vi "Deserialisierer.vi"(9 "Enum":T3(ring), 11 "CAN Daten":T1[](array[typedef]) {"payload" format="%x"; "timestamp" format="%<%.7X\n%x>T"; "type" items=["CAN Data"=0, "CAN Remote"=1, "CAN Bus Error"=2, "CAN 2.0 Data"=8, "CAN FD Data"=16, "CAN FD+BRS Data"=24, "J1939 Data"=192, "Delay"=224, "Log Trigger"=225, "Start Trigger"=226]; "identifier" format="%x"}) -> (1 "Output":sgl[](array[numeric]), 3 "identifier":u32)   [LabVIEW 2020, in "CAN Interface.lvlib"]
uses:
  CAN Interface.lvlib
  <vilib>/xnet/xnet.llb/XNET Frame CAN.ctl
  <vilib>/xnet/xnet.llb/XNET Frame Type CAN.ctl
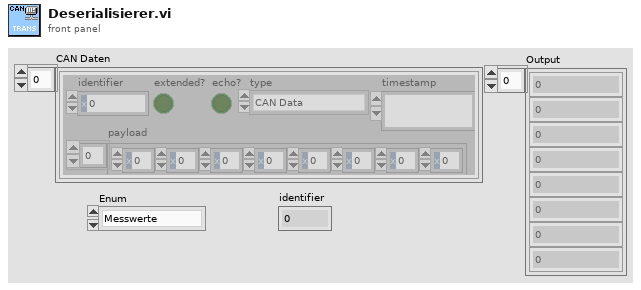
[diagram p1: front panel]
types:
  T1 = typedef "XNET Frame CAN.ctl" = cluster{"timestamp":timestamp, "payload":u8[], "identifier":u32, "type":T2, "extended?":bool, "echo?":bool}
  T2 = typedef "XNET Frame Type CAN.ctl" = u8
  T3 = enum16{"Messwerte", "Fluss, Druck", "Temperaturen 1", "Temperaturen 2", "Fehler", "Zustand, spülen?"}
  T4 = enum16{"big-endian, network order", "native, host order", "little-endian"}
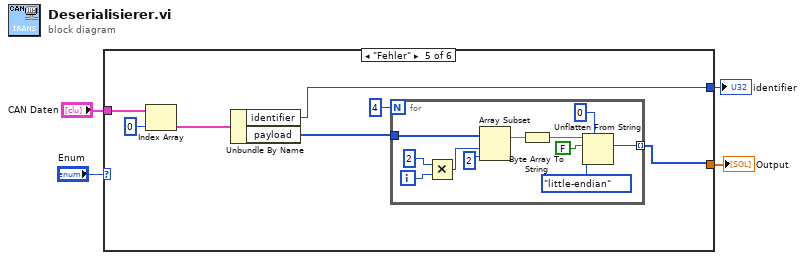
[diagram p0: block diagram]
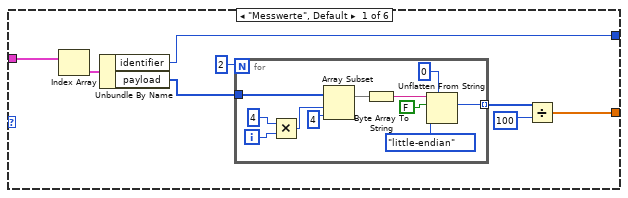
[diagram p2: hidden frame]
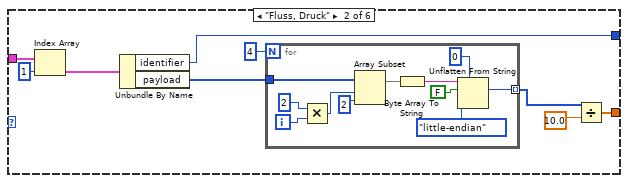
[diagram p3: hidden frame]
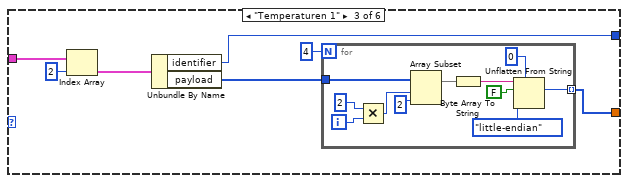
[diagram p4: hidden frame]
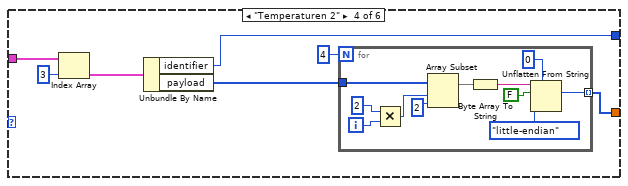
[diagram p5: hidden frame]
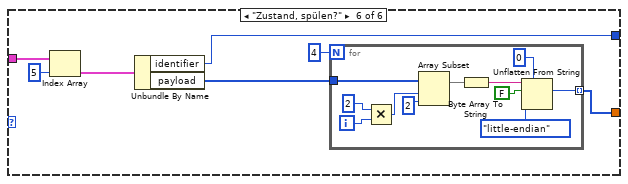
[diagram p6: hidden frame]
diagram:
  n1 = case shown="\"Fehler\"" "Enum" {
    tunnel: [w7 w27 w44 w63 w83 w98] -> w2
    tunnel: "CAN Daten" -> [w6 w29 w46 w64 w84 w100]
    tunnel: [w5 w25 w45 w62 w81 w99] -> w1
    frame "Messwerte", Default {
      n2 = Index Array(array=w6) -> (element=w8:T1)  [unwired: 1 in]
      n3 = Unbundle By Name(w8) -> ("identifier"=w7:u32, "payload"=w9:u8[])
      n4 = for {
        N: 2 -> [_]
        tunnel: w9 -> [w20]
        tunnel: [w13] -> w12 mode=indexing
        i -> [w23]
        n5 = Multiply(x=4, y=w23) -> (x*y=w21:i32)
        n6 = Array Subset(array=w20, index=w21, length=4 ("Länge")) -> (w14:u8[])
        n7 = Byte Array To String(unsigned byte array=w14) -> (string=w15:string)
        n8 = Unflatten From String(type=i16 0, binary string=w15, data includes array or string size? (T)=FALSE ("Enthält Array- oder String-Größe? (T)"), byte order (0:big-endian, network order)=T4."little-endian" ("Byte-Reihenfolge (0:Big-Endian, Netzwerkreihenfolge)")) -> (value=w13:i16)  [unwired: 1 in, 2 out]
      }
      n9 = Divide(x=w12, y=i16 100) -> (x/y=w5:dbl[])
    }
    frame "Fluss, Druck" {
      n10 = Index Array(array=w29, index=1 ("Index")) -> (element=w30:T1)
      n11 = Unbundle By Name(w30) -> ("identifier"=w27:u32, "payload"=w31:u8[])
      n12 = for {
        N: 4 -> [_]
        tunnel: w31 -> [w40]
        tunnel: [w33] -> w24 mode=indexing
        i -> [w43]
        n13 = Multiply(x=2, y=w43) -> (x*y=w41:i32)
        n14 = Array Subset(array=w40, index=w41, length=2 ("Länge")) -> (w34:u8[])
        n15 = Byte Array To String(unsigned byte array=w34) -> (string=w35:string)
        n16 = Unflatten From String(type=u16 0, binary string=w35, data includes array or string size? (T)=FALSE ("Enthält Array- oder String-Größe? (T)"), byte order (0:big-endian, network order)=T4."little-endian" ("Byte-Reihenfolge (0:Big-Endian, Netzwerkreihenfolge)")) -> (value=w33:u16)  [unwired: 1 in, 2 out]
      }
      n17 = Divide(x=w24, y=sgl 10.0) -> (x/y=w25:sgl[])
    }
    frame "Temperaturen 1" {
      n18 = Index Array(array=w46, index=2 ("Index")) -> (element=w48:T1)
      n19 = Unbundle By Name(w48) -> ("identifier"=w44:u32, "payload"=w49:u8[])
      n20 = for {
        N: 4 -> [_]
        tunnel: w49 -> [w58]
        tunnel: [w51] -> w45 mode=indexing
        i -> [w61]
        n21 = Multiply(x=2, y=w61) -> (x*y=w59:i32)
        n22 = Array Subset(array=w58, index=w59, length=2 ("Länge")) -> (w52:u8[])
        n23 = Byte Array To String(unsigned byte array=w52) -> (string=w53:string)
        n24 = Unflatten From String(type=i16 0, binary string=w53, data includes array or string size? (T)=FALSE ("Enthält Array- oder String-Größe? (T)"), byte order (0:big-endian, network order)=T4."little-endian" ("Byte-Reihenfolge (0:Big-Endian, Netzwerkreihenfolge)")) -> (value=w51:i16)  [unwired: 1 in, 2 out]
      }
    }
    frame "Temperaturen 2" {
      n25 = Index Array(array=w64, index=3 ("Index")) -> (element=w66:T1)
      n26 = Unbundle By Name(w66) -> ("identifier"=w63:u32, "payload"=w67:u8[])
      n27 = for {
        N: 4 -> [_]
        tunnel: w67 -> [w76]
        tunnel: [w69] -> w62 mode=indexing
        i -> [w79]
        n28 = Multiply(x=2, y=w79) -> (x*y=w77:i32)
        n29 = Array Subset(array=w76, index=w77, length=2 ("Länge")) -> (w70:u8[])
        n30 = Byte Array To String(unsigned byte array=w70) -> (string=w71:string)
        n31 = Unflatten From String(type=i16 0, binary string=w71, data includes array or string size? (T)=FALSE ("Enthält Array- oder String-Größe? (T)"), byte order (0:big-endian, network order)=T4."little-endian" ("Byte-Reihenfolge (0:Big-Endian, Netzwerkreihenfolge)")) -> (value=w69:i16)  [unwired: 1 in, 2 out]
      }
    }
    frame "Fehler" {
      n32 = Index Array(array=w84, index=0 ("Index")) -> (element=w86:T1)
      n33 = Unbundle By Name(w86) -> ("identifier"=w83:u32, "payload"=w80:u8[])
      n34 = for {
        N: 4 -> [_]
        tunnel: w80 -> [w94]
        tunnel: [w87] -> w81 mode=indexing
        i -> [w97]
        n35 = Multiply(x=2, y=w97) -> (x*y=w95:i32)
        n36 = Array Subset(array=w94, index=w95, length=2 ("Länge")) -> (w88:u8[])
        n37 = Byte Array To String(unsigned byte array=w88) -> (string=w89:string)
        n38 = Unflatten From String(type=i16 0, binary string=w89, data includes array or string size? (T)=FALSE ("Enthält Array- oder String-Größe? (T)"), byte order (0:big-endian, network order)=T4."little-endian" ("Byte-Reihenfolge (0:Big-Endian, Netzwerkreihenfolge)")) -> (value=w87:i16)  [unwired: 1 in, 2 out]
      }
    }
    frame "Zustand, spülen?" {
      n39 = Index Array(array=w100, index=5 ("Index")) -> (element=w103:T1)
      n40 = Unbundle By Name(w103) -> ("identifier"=w98:u32, "payload"=w102:u8[])
      n41 = for {
        N: 4 -> [_]
        tunnel: w102 -> [w112]
        tunnel: [w105] -> w99 mode=indexing
        i -> [w115]
        n42 = Multiply(x=2, y=w115) -> (x*y=w113:i32)
        n43 = Array Subset(array=w112, index=w113, length=2 ("Länge")) -> (w106:u8[])
        n44 = Byte Array To String(unsigned byte array=w106) -> (string=w107:string)
        n45 = Unflatten From String(type=i16 0, binary string=w107, data includes array or string size? (T)=FALSE ("Enthält Array- oder String-Größe? (T)"), byte order (0:big-endian, network order)=T4."little-endian" ("Byte-Reihenfolge (0:Big-Endian, Netzwerkreihenfolge)")) -> (value=w105:i16)  [unwired: 1 in, 2 out]
      }
    }
  }
  "identifier" <- w2
  "Output" <- w1
